vi "Create Grid.vi"(5 "Color":u32(colorbox), 7 "Style":T2, 8 "error in (no error)":errorcluster, 9 "Draw Area":T1, 10 "Horizontal Step":i32, 11 "Vertical Step":i32) -> (0 "error out":errorcluster, 3 "Grid Reference":refnum<data-value>)   [LabVIEW 2017, in "LV Image Editor Framework.lvlib" / "Grid.lvclass"]
uses:
  Grid.lvclass
  Shape/Shape.lvclass
  <vilib>/Utility/miscctls.llb/LVBoundsTypeDef.ctl
  C:/Github/LIEF/Forms/Shape/Shape.lvclass
  Shape/Shape.lvclass/Shape.ctl
  Line/Line.lvclass/Line.ctl
  Grid.lvclass/Grid.ctl
  Shape/Write Color.vi
  Line/Write Style.vi
  Line/Line.lvclass
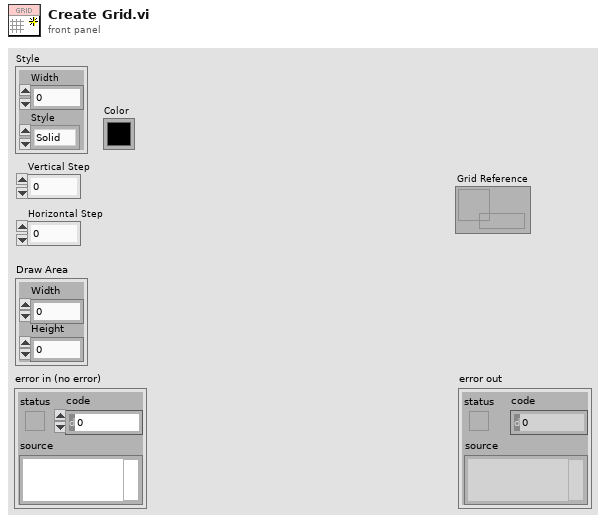
[diagram p1: front panel]
types:
  T1 = typedef "LVBoundsTypeDef.ctl" = cluster{"Width":u32, "Height":u32}
  T2 = cluster{"Width":u16, "Style":enum32{"Solid", "Dash", "Dot", "DashDot", "DashDotDot"}}
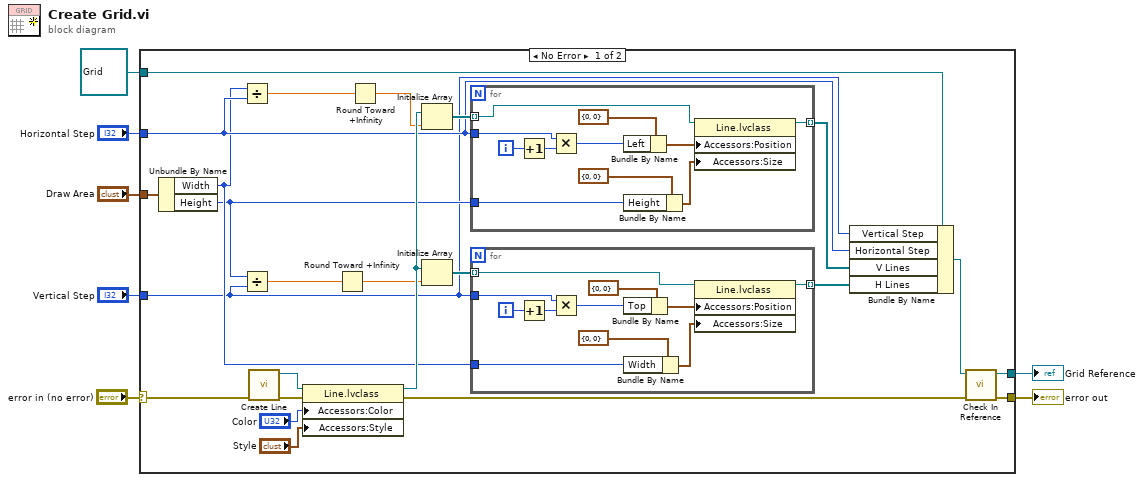
[diagram p0: block diagram]
diagram:
  n1 = case shown="No Error" "error in (no error)" {
    selector: "error in (no error)" -> [w11 w54]
    tunnel: [w9 w54] -> w6
    tunnel: refnum<class "Grid.lvclass"> refnum ("Grid in") -> [w26 _]
    tunnel: [w31 _] -> w4
    tunnel: "Vertical Step" -> [w13 _]
    tunnel: "Horizontal Step" -> [w19 _]
    tunnel: "Draw Area" -> [w23 _]
    frame No Error {
      n2 = Unbundle By Name(w23) -> ("Width"=w16:u32, "Height"=w14:u32)
      n3 = Divide(x=w16, y=w19) -> (x/y=w22:dbl)
      n4 = Divide(x=w14, y=w13) -> (x/y=w15:dbl)
      n5 = call "Create Line.vi"("error in (no error)"=w11) -> ("error out"=w30:errorcluster, "Line out"=w29:refnum<class "Line.lvclass">)  [unwired: 9 in]
      n6 = property class="Line.lvclass"(reference=w29, error in=w30, "Accessors:Color"="Color", "Accessors:Style"="Style") -> (reference out=w24:refnum<class "Line.lvclass">, error out=w10:errorcluster)
      n7 = Round Toward +Infinity(x=w15) -> (ceil(x): smallest int >= x=w8:dbl)
      n8 = Round Toward +Infinity(x=w22) -> (ceil(x): smallest int >= x=w21:dbl)
      n9 = Initialize Array(w24, w21) -> (w20:refnum<class "Line.lvclass">[])
      n10 = Initialize Array(w24, w8) -> (w17:refnum<class "Line.lvclass">[])
      n11 = for {
        tunnel: w20 -> [w53] mode=indexing
        tunnel: w19 -> [w50]
        tunnel: w14 -> [w44]
        tunnel: [w43] -> w18 mode=indexing
        i -> [w52]
        n12 = Increment(x=w52) -> (x+1=w51:i32)
        n13 = Multiply(x=w50, y=w51) -> (x*y=w48:i32)
        n14 = Bundle By Name(cluster=cluster{"Left":i32, "Top":i32} {"Left"=0, "Top"=0} ("Position"), "Left"=w48) -> (w47:cluster{"Left":i32, "Top":i32})
        n15 = Bundle By Name(cluster=cluster{"Width":i32, "Height":i32} {"Width"=0, "Height"=0} ("Size"), "Height"=w44) -> (w45:cluster{"Width":i32, "Height":i32})
        n16 = property class="Line.lvclass"(reference=w53, "Accessors:Position"=w47, "Accessors:Size"=w45) -> (reference out=w43:refnum<class "Line.lvclass">)  [unwired: 1 in, 1 out]
      }
      n17 = for {
        tunnel: w17 -> [w42] mode=indexing
        tunnel: w13 -> [w39]
        tunnel: w16 -> [w33]
        tunnel: [w32] -> w12 mode=indexing
        i -> [w41]
        n18 = Increment(x=w41) -> (x+1=w40:i32)
        n19 = Multiply(x=w39, y=w40) -> (x*y=w37:i32)
        n20 = Bundle By Name(cluster=cluster{"Left":i32, "Top":i32} {"Left"=0, "Top"=0} ("Position"), "Top"=w37) -> (w36:cluster{"Left":i32, "Top":i32})
        n21 = Bundle By Name(cluster=cluster{"Width":i32, "Height":i32} {"Width"=0, "Height"=0} ("Size"), "Width"=w33) -> (w34:cluster{"Width":i32, "Height":i32})
        n22 = property class="Line.lvclass"(reference=w42, "Accessors:Position"=w36, "Accessors:Size"=w34) -> (reference out=w32:refnum<class "Line.lvclass">)  [unwired: 1 in, 1 out]
      }
      n23 = Bundle By Name(cluster=w26, "Vertical Step"=w13, "Horizontal Step"=w19, "V Lines"=w18, "H Lines"=w12) -> (w25:refnum<class "Grid.lvclass">)
      n24 = call "Check In Reference.vi"("error in (no error)"=w10, "Shape in"=w25) -> ("error out"=w9:errorcluster, "Shape Reference"=w31:refnum<data-value>)  [unwired: 8 in]
    }
    frame Error {
    }
  }
  "error out" <- w6
  "Grid Reference" <- w4
